vi "set_inlet_blockage.vi"(6 "timeout (25000ms)":i32=25000, 8 "error in (no error)":errorcluster, 10 "rpm":i32, 11 "daemon reference in":refnum<k5>) -> (0 "error out":errorcluster, 2 "response":string, 3 "daemon reference out":refnum<k5>, 5 "command out":string="random")   [LabVIEW 2017]
doc: "<b>Command: </b>\"set_inlet_blockage\"\n\n<b>Description: </b> This command is to calibrate inlte blockage derate during eol. Set -1 to clear existing setting, set 0 to start auto calibration when motor running in steady mode.\n\n<b>Parameters: </b> speed in rpm\n____________________________________________\nDIPC 692 Daemon API 10.0.0.1\nSam Tee - Dyson Technology Ltd\nCopyright (c) 2024, Dyson Technology Ltd"
panel:
  out "parameter(s) in":string
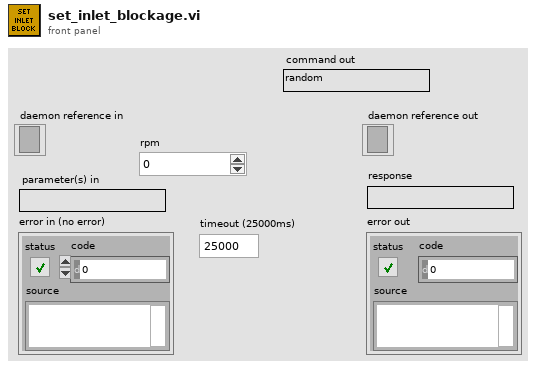
[diagram p1: front panel]
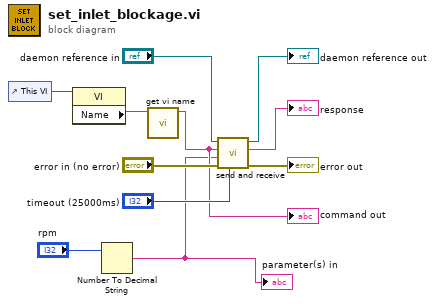
[diagram p0: block diagram]
diagram:
  n1 = control-ref of="This VI"() -> (w5:refnum<vi>)
  n2 = property class="VI"(reference=w5) -> ("Name"=w4:string)  [unwired: 1 in, 2 out]
  n3 = Number To Decimal String(number="rpm") -> (decimal integer string=w1:string)  [unwired: 1 in]
  "parameter(s) in" <- w1
  n4 = call "get vi name.vi"("library.lvlib:name.vi"=w4) -> ("vi name"=w3:string)  [unwired: 10 in]
  "command out" <- w3
  n5 = call "send and receive.vi"("timeout (25000ms)"="timeout (25000ms)", "error in (no error)"="error in (no error)", "data"=w1, "command"=w3, "daemon reference in"="daemon reference in") -> ("error out"=→"error out":errorcluster, "response"=→"response":string, "daemon reference out"=→"daemon reference out":refnum<k5>)  [unwired: 4 in]
